vi "Configure Channel (DI Pulse).vi"(0 "VISA resource name":refnum<visa-resource-name>, 5 "Channel (0001)":string="0001", 7 "Enable Channel (True)":bool=TRUE, 9 "Span":T1={"Lower Span (0)"=0, "Upper Span (1250)"=1250} {"Upper Span (1250)" min=0 max=999999 step=1; "Lower Span (0)" min=-99999 max=99999 step=1}, 11 "error in (no error)":errorcluster) -> (4 "VISA resource name out":refnum<visa-resource-name>, 6 "Channel":string, 15 "error out":errorcluster)   [LabVIEW 2020, in "Yokogawa GX Series.lvlib"]
doc: "Sets the input range of DI channels in pulse input.\n\nCommand: SRangeDI"
uses:
  <instrlib>/Yokogawa GX Series/Yokogawa GX Series.lvlib
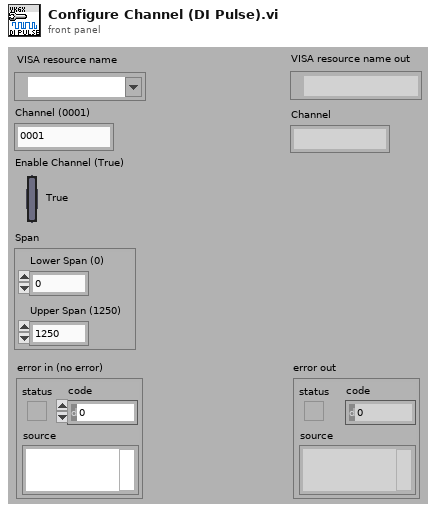
[diagram p1: front panel]
types:
  T1 = cluster{"Lower Span (0)":i32, "Upper Span (1250)":i32}
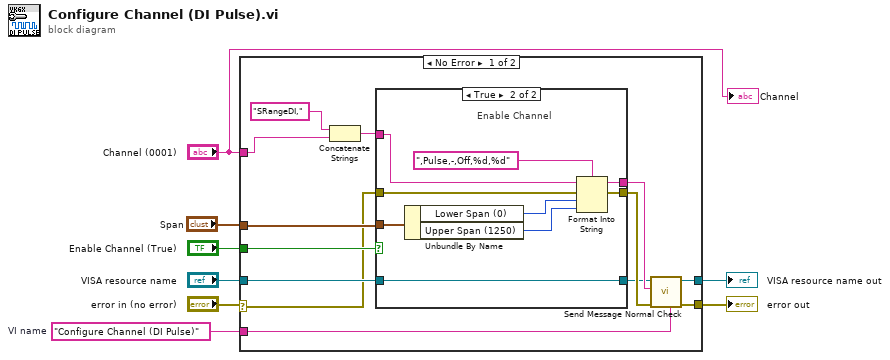
[diagram p0: block diagram]
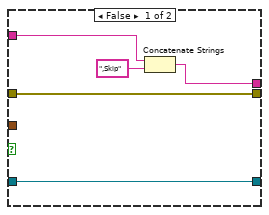
[diagram p2: hidden frame]
diagram:
  w5 = "Configure Channel (DI Pulse)"  # VI name
  n1 = case shown="No Error" "error in (no error)" {
    selector: "error in (no error)" -> [w12 w36]
    tunnel: "Enable Channel (True)" -> [w21 _]
    tunnel: [w20 w37] -> w7
    tunnel: [w19 w36] -> w6
    tunnel: w5 -> [w16 _]
    tunnel: "Span" -> [w15 _]
    tunnel: "VISA resource name" -> [w14 w37]
    tunnel: "Channel (0001)" -> [w9 _]
    frame No Error {
      n2 = Concatenate Strings("SRangeDI,", w9) -> (w11:string)
      n3 = case shown="True" w21 {
        tunnel: w12 -> [w23 w34]
        tunnel: [w23 w33] -> w18
        tunnel: w11 -> [w24 w27]
        tunnel: [w25 w32] -> w17
        tunnel: w15 -> [_ w31]
        tunnel: w14 -> [w22 w30]
        tunnel: [w22 w30] -> w13
        frame False {
          n4 = Concatenate Strings(w24, ",Skip") -> (w25:string)
        }
        frame True {
          # "Enable Channel"
          n5 = Unbundle By Name(w31) -> ("Lower Span (0)"=w29:i32, "Upper Span (1250)"=w28:i32)
          n6 = Format Into String(format string=",Pulse,-,Off,%d,%d", initial string=w27, error in=w34, w29, w28) -> (resulting string=w32:string, error out=w33:errorcluster)
        }
      }
      n7 = call <instrlib>:"Send Message Normal Check.vi"("Source (\"\")"=w16, "error in (no error)"=w18, "Send Message (\"\")"=w17, "VISA resource name"=w13) -> ("error out"=w19:errorcluster, "VISA resource name out"=w20:refnum<visa-resource-name>)  [unwired: 2 in, 4 out]
    }
    frame Error {
    }
  }
  "error out" <- w6
  "VISA resource name out" <- w7
  "Channel" <- "Channel (0001)"
